vi "CALC_MATH_MEM.vi"(0 "VISA IN":refnum<visa-resource-name>, 5 "error in":errorcluster, 7 "Channel":i32) -> (14 "VISA Out":refnum<visa-resource-name>, 19 "error out":errorcluster)   [LabVIEW 2018, in "PNA-X.lvlib"]
doc: "CALCulate<cnum>:MATH:MEMorize \n(Write-only) Puts the currently selected measurement trace into memory. (Data-> Memory). \nSee Critical Note \nParameters \n<cnum> Channel number of the measurement. There must be a selected measurement \non that channel. If unspecified, <cnum> is set to 1. \nExamples CALC:MATH:MEM \ncalculate2:math:memorize \nQuery Syntax Not applicable \nDefault Not applicable \n1545\n\nCalculate:Mixer Command \nCALCulate<ch>:MIXer:XAXis <char> \n(Read-Write) Sets or returns the swept parameter to display on the X-axis for the selected FCA \nmeasurement. Learn more about X-axis display. \nCritical Note: CALCulate commands act on the selected measurement. You can select one \nmeasurement for each channel using Calc:Par:Select \nParameters \n<ch> Any existing channel number. If unspecified, value is set to 1. \n<char> Parameter to display on the X-axis. Choose from: \nINPUT - Input frequency span \nOUTPUT - Output frequency span \nLO_1 - First LO frequency span \nLO_2 - Second LO frequency span \nExamples CALC:MIX:XAX INPUT \ncalc2:mixer:xaxis output \nSee an example that creates, selects, and calibrates an SMC and \nVMC measurement using SCPI. \nQuery Syntax CALCulate<ch>:MIXer:XAXis? \nReturn Type Character \nDefault OUTPUT \n1546\n\nCalculate:Normalize Commands \nSpecifies the normalization features used for a receiver power calibration. \nThese commands are Superseded (Sept 2004). \nSee the replacement commands in a new Receiver Power Cal example. \nClick on a blue keyword to view the command details. \nSee Also \nExample Programs \nLearn about Receiver Cal \nSCPI Command Tree \nSave and recall your receiver power calibration (which use .CST file commands): \nSENS:CORR:CSET:SAVE \nSENS:CORR:CSET[:SEL] \nOr use these two commands and specify either .STA or .CST file extensions: \nMMEM:LOAD \nMMEM:STOR \nCritical Note: CALCulate commands act on the selected measurement. You can select one \nmeasurement for each channel using Calc:Par:Select"
uses:
  PNA-X.lvlib
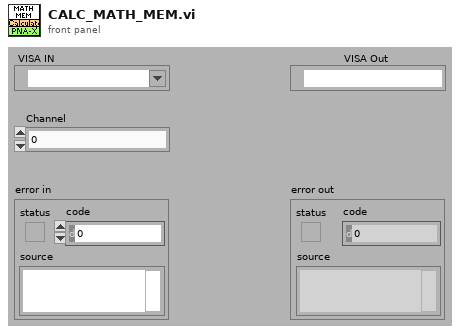
[diagram p1: front panel]
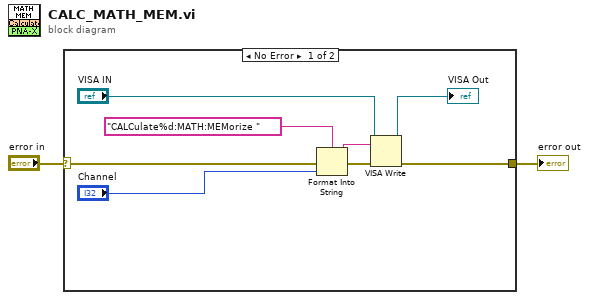
[diagram p0: block diagram]
diagram:
  n1 = case shown="No Error" "error in" {
    selector: "error in" -> [w10 w11]
    tunnel: [w5 w11] -> w1
    frame No Error {
      n2 = Format Into String(format string="CALCulate%d:MATH:MEMorize " ("Cmdline"), error in=w10, "Channel") -> (resulting string=w8:string, error out=w9:errorcluster)  [unwired: 1 in]
      n3 = VISA Write(VISA resource name="VISA IN", write buffer=w8, error in (no error)=w9) -> (VISA resource name out=→"VISA Out":refnum<visa-resource-name>, error out=w5:errorcluster)  [unwired: 1 out]
    }
    frame Error {
    }
  }
  "error out" <- w1
